vi "GetVisionFiringBox.vi"   [LabVIEW 2015]
uses:
  Robot Global Data.vi
types:
  T1 = cluster{"Angle":dbl, "Distance":dbl, "x":dbl, "y":dbl}
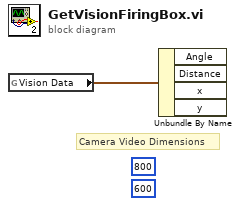
[diagram p0: block diagram]
diagram:
  (unwired) 600
  (unwired) 800
  # "Camera Video Dimensions"
  n1 = global read "Robot Global Data.vi" "Vision Data"() -> (w1:T1)
  n2 = Unbundle By Name(w1) -> ()  [unwired: 4 out]
